vi "AutoWait.vi"(1 "Time Since Latch":u32, 2 "Instruction String":string) -> (0 "Advance Trigger":bool)   [LabVIEW 2018]
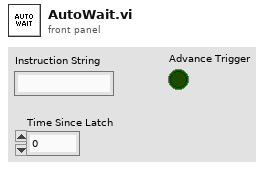
[diagram p1: front panel]
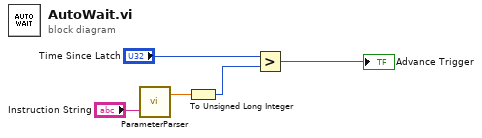
[diagram p0: block diagram]
diagram:
  n1 = call "ParameterParser.vi"("Parameter String"="Instruction String") -> ("Parameter"=w2:dbl)  [unwired: 1 in, 1 out]
  n2 = To Unsigned Long Integer(number=w2) -> (unsigned 32bit integer=w1:u32)
  n3 = Greater?(x="Time Since Latch", y=w1) -> (0:→"Advance Trigger":bool)
